vi "Read XY.vi"(8 "error in (no error)":errorcluster, 11 "Element in":refnum<class "Element.lvclass">) -> (0 "error out":errorcluster, 2 "XY":cluster{"X":i32[], "Y":i32[]}, 3 "Element out":refnum<class "Element.lvclass">)   [LabVIEW 2019, in "Element.lvclass"]
uses:
  Element.lvclass
  Element.lvclass/Element.ctl
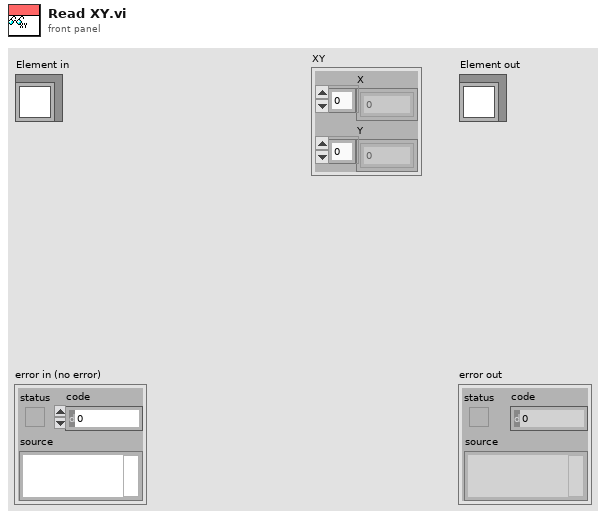
[diagram p1: front panel]
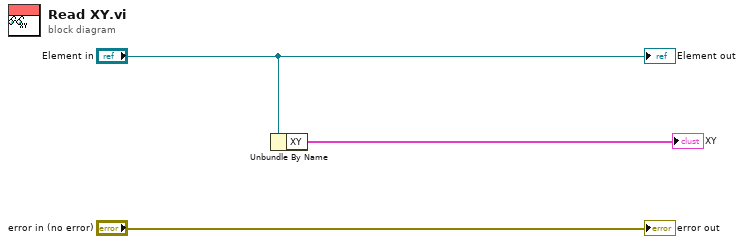
[diagram p0: block diagram]
diagram:
  n1 = Unbundle By Name("Element in") -> ("XY"=→"XY":cluster{"X":i32[], "Y":i32[]})
  "error out" <- "error in (no error)"
  "Element out" <- "Element in"
